vi "Finalize Turn Check.vi"(7 "Actor in":refnum<class "Actor.lvclass">, 8 "Error in":errorcluster) -> (0 "Error out":errorcluster, 2 "Proceed To Tearing Down":bool, 5 "Actor out":refnum<class "Actor.lvclass">)   [LabVIEW 2020, in "jettl.lvlib"]
uses:
  jettl.lvlib
  Actor/Actor.lvclass
  Msg/Msg.lvclass
  Lifetime.ctl
  Stop jettl Msg/Stop/Stop.lvlib
  Stopping jettl Msg/Stopping/Stopping.lvlib
  Stopping jettl Msg/Stopping/Tell Parent.vi
  Stopping jettl Msg/Stopping/Tell Child.vi
  Stop jettl Msg/Stop/Tell Self.vi
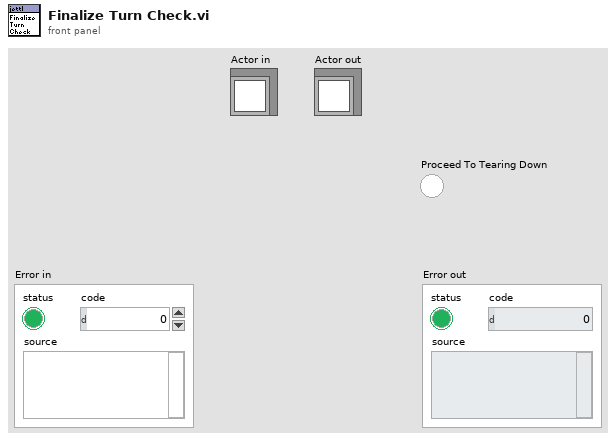
[diagram p1: front panel]
types:
  T1 = typedef "jettl.lvlib/Lifetime.ctl" = enum16{"Init", "Spawn", "Setup", "Teardown Before Running", "Running", "Stop Called", "Stopping With Children", "Stopping Without Children", "Teardown After Running", "Stopped"}
  T2 = typedef "jettl.lvlib/Child Aliases.ctl" = set{string}
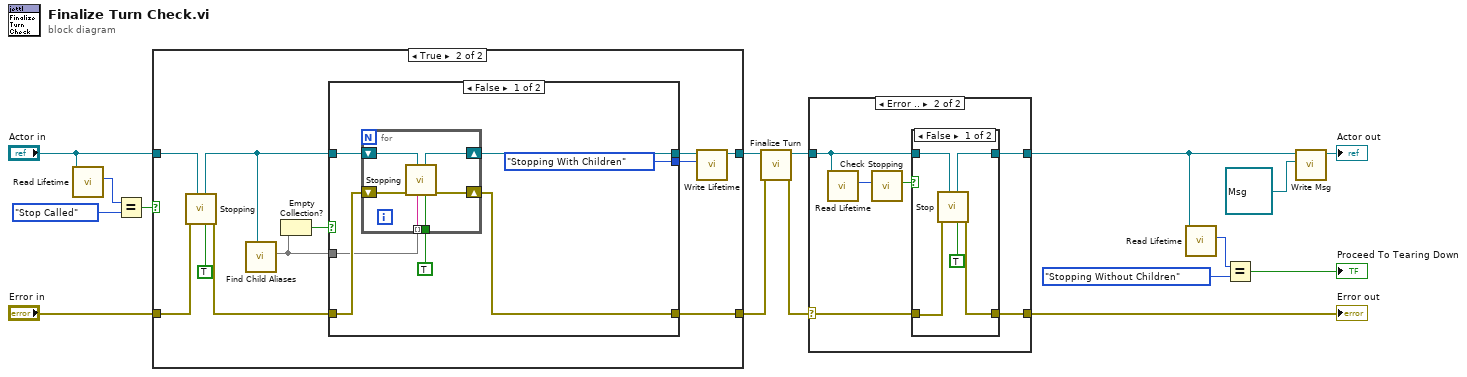
[diagram p0: block diagram]
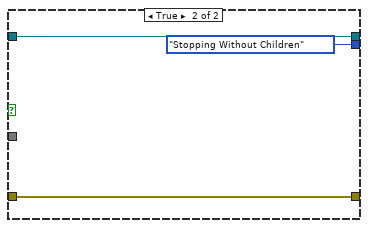
[diagram p3: hidden frame]
diagram:
  n1 = call-dynamic "Read Lifetime.vi"("Actor in"="Actor in") -> ("Lifetime"=w7:T1)  [unwired: 10 in]
  n2 = Equal?(x=w7, y=Lifetime."Stop Called") -> (x = y?=w5:bool)
  n3 = case shown="True" w5 {
    tunnel: "Error in" -> [w18 w24]
    tunnel: [w18 w29] -> w3
    tunnel: [w17 w21] -> w1
    tunnel: "Actor in" -> [w17 w26]
    frame False {
    }
    frame True {
      n4 = call-poly "Stopping.vi"("Priority"=TRUE, "Actor in"=w26, "Error in"=w24) -> ("Error out"=w23:errorcluster, "Actor out"=w25:refnum<class "Actor.lvclass">)  [unwired: 7 in]
      n5 = call "Find Child Aliases.vi"("Actor in"=w25) -> ("Child Aliases"=w28:T2)  [unwired: 10 in]
      n6 = Empty Collection?(1:w28) -> (0:w27:bool)
      n7 = case shown="False" w27 {
        tunnel: w23 -> [w36 w43]
        tunnel: [w35 w43] -> w29
        tunnel: [Lifetime."Stopping With Children" ("Lifetime") Lifetime."Stopping Without Children" ("Lifetime")] -> w20
        tunnel: w25 -> [w34 w44]
        tunnel: [w33 w44] -> w22
        tunnel: w28 -> [w32 _]
        frame False {
          n8 = for {
            tunnel: w32 -> [w42] mode=indexing
            shift-right: [w40] -> w35
            shift-left: w36 -> [w41]
            shift-right: [w38] -> w33
            shift-left: w34 -> [w39]
            tunnel: TRUE ("Priority") -> [w37]
            n9 = call-poly "Stopping.vi"("Priority"=w37, "Alias"=w42, "Actor in"=w39, "Error in"=w41) -> ("Error out"=w40:errorcluster, "Actor out"=w38:refnum<class "Actor.lvclass">)  [unwired: 6 in]
          }
        }
        frame True {
        }
      }
      n10 = call-dynamic "Write Lifetime.vi"("Lifetime"=w20, "Actor in"=w22) -> ("Actor out"=w21:refnum<class "Actor.lvclass">)  [unwired: 9 in]
    }
  }
  n11 = call-dynamic "Finalize Turn.vi"("Error in"=w3, "Actor in"=w1) -> ("Error out"=w11:errorcluster, "Actor out"=w10:refnum<class "Actor.lvclass">)  [unwired: 8 in]
  n12 = case shown="Error .." w11 {
    selector: w11 -> [_ w50]
    tunnel: [w46 w52] -> w9
    tunnel: [_ w51] -> w8
    tunnel: w10 -> [w46 w49]
    frame No Error {
    }
    frame Error {
      n13 = call-dynamic "Read Lifetime.vi"("Actor in"=w49) -> ("Lifetime"=w48:T1)  [unwired: 10 in]
      n14 = call "Check Stopping.vi"("Lifetime"=w48) -> ("Stopping"=w47:bool)  [unwired: 10 in]
      n15 = case shown="False" w47 {
        tunnel: [w56 w59] -> w52
        tunnel: w49 -> [w57 w59]
        tunnel: w50 -> [w55 w58]
        tunnel: [w54 w58] -> w51
        frame False {
          n16 = call-poly "Stop.vi"("Priority"=TRUE, "Actor in"=w57, "Error in"=w55) -> ("Error out"=w54:errorcluster, "Actor out"=w56:refnum<class "Actor.lvclass">)  [unwired: 7 in]
        }
        frame True {
        }
      }
    }
  }
  "Error out" <- w8
  n17 = call-dynamic "Read Lifetime.vi"("Actor in"=w9) -> ("Lifetime"=w16:T1)  [unwired: 10 in]
  n18 = Equal?(x=w16, y=Lifetime."Stopping Without Children") -> (x = y?=→"Proceed To Tearing Down":bool)
  n19 = call-dynamic "Write Msg.vi"("Msg"=refnum<class "Msg.lvclass"> refnum, "Actor in"=w9) -> ("Actor out"=→"Actor out":refnum<class "Actor.lvclass">)  [unwired: 9 in]
